vi "Read Waveform Measurement Two Channel.vi"(5 "Channel B (2: Channel 2)":u16(ring)=2 items=["Channel 1"=1, "Channel 2"=2, "Channel 3"=3, "Channel 4"=4], 6 "Measurement Function (0: Falling Edge)":u16(ring) items=["VRatio(Display)", "VRatio(Cycle)", "Raising Edge Delay", "Falling Edge Delay", "Raising to Falling Edge Delay", "Falling to Raising Edge Delay", "Raising Edge Phase", "Falling Edge Phase"], 7 "Channel A(1: Channel 1)":u16(ring)=1 items=["Channel 1"=1, "Channel 2"=2, "Channel 3"=3, "Channel 4"=4], 8 "error in (no error)":errorcluster, 9 "Measurement Type (0: Statistic Average)":u16(ring) items=["Statistic Average", "Current Statistic Value", "Statistic Maximum", "Statistic Minimum", "Statistic Standard Deviation", "Counter"], 10 "Timeout (1000 ms)":dbl=1000.0, 11 "VISA resource name":refnum<visa-resource-name>) -> (0 "error out":errorcluster, 2 "Measurement":dbl, 3 "VISA resource name out":refnum<visa-resource-name>)   [LabVIEW 2015, in "ZhiYuan ZDS Series for TCP.lvlib"]
doc: "Returns the waveform the oscilloscope acquired for the specified channel. The waveform is from an acquisition that you initiate prior to calling this VI.\n\nYou use the Initiate VI to start an acquisition on the channels that you enable with the Configure Channel VI. The oscilloscope acquires waveforms for the enabled channels concurrently. You must call this VI separately for each enabled channel to obtain the waveforms.\n\nYou can call the Read Waveform VI instead of using low-level VIs.\n\n<B>Note:</B> Use this VI only with other low-level VIs. The high-level VIs automatically incorporate this functionality. This VI does not check the instrument status."
uses:
  ZhiYuan ZDS Series for TCP.lvlib
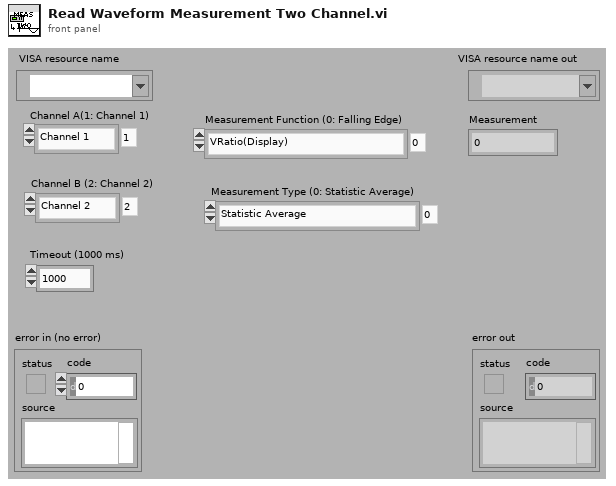
[diagram p1: front panel]
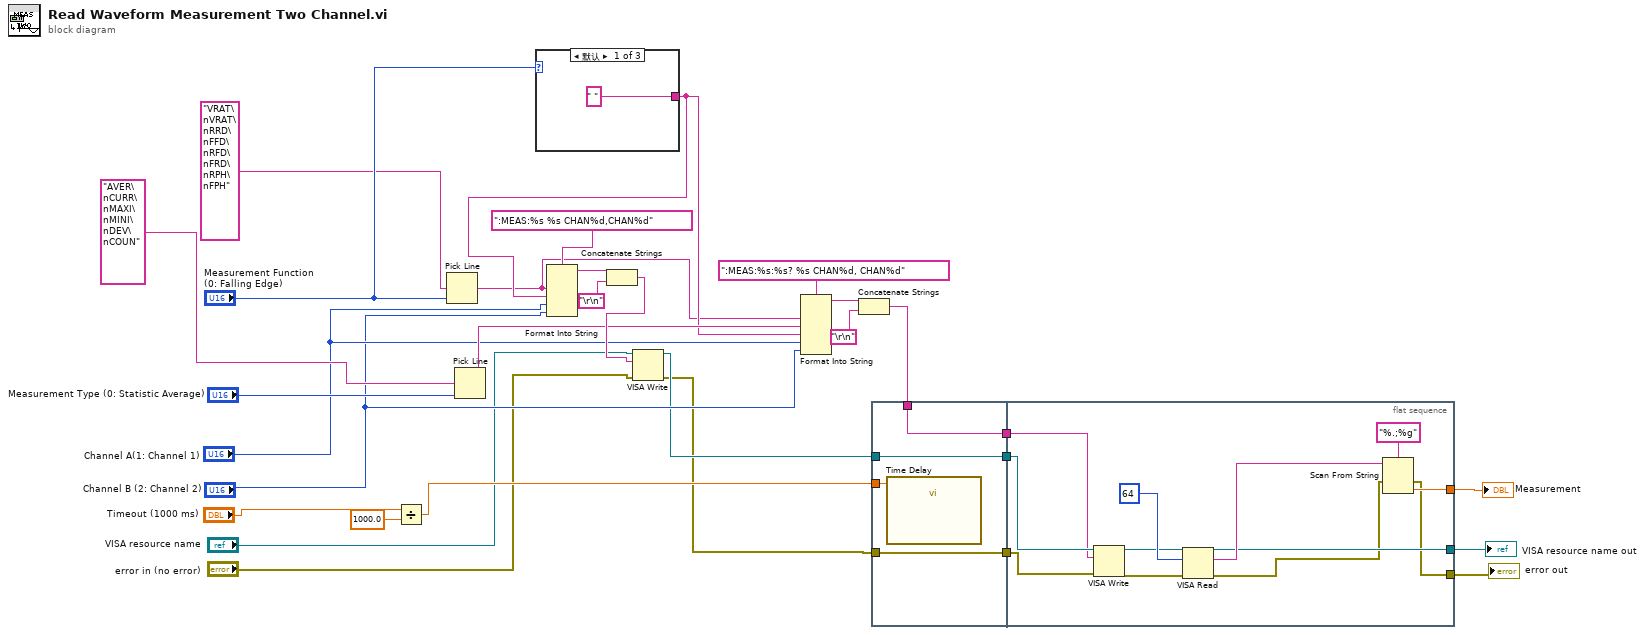
[diagram p0: block diagram]
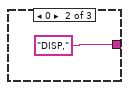
[diagram p2: hidden frame]
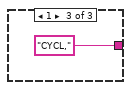
[diagram p3: hidden frame]
diagram:
  n1 = Divide(x="Timeout (1000 ms)", y=1000.0) -> (x/y=w10:dbl)
  n2 = Pick Line(multi-line string="VRAT\nVRAT\nRRD\nFFD\nRFD\nFRD\nRPH\nFPH", line index="Measurement Function (0: Falling Edge)") -> (output string=w1:string)  [unwired: 1 in]
  n3 = Pick Line(multi-line string="AVER\nCURR\nMAXI\nMINI\nDEV\nCOUN", line index="Measurement Type (0: Statistic Average)") -> (output string=w19:string)  [unwired: 1 in]
  n4 = case shown="默认" "Measurement Function (0: Falling Edge)" {
    tunnel: [" " "DISP," "CYCL,"] -> w18
    frame Default {
    }
    frame 0 {
    }
    frame 1 {
    }
  }
  n5 = Format Into String(format string=":MEAS:%s %s CHAN%d,CHAN%d" ("write buffer"), w1, w18, "Channel A(1: Channel 1)", "Channel B (2: Channel 2)") -> (resulting string=w24:string)  [unwired: 2 in, 1 out]
  n6 = Concatenate Strings(w24, "\r\n") -> (w22:string)
  n7 = VISA Write(VISA resource name="VISA resource name", write buffer=w22, error in (no error)="error in (no error)") -> (VISA resource name out=w3:refnum<visa-resource-name>, error out=w2:errorcluster)  [unwired: 1 out]
  n8 = Format Into String(format string=":MEAS:%s:%s? %s CHAN%d, CHAN%d", w1, w19, w18, "Channel A(1: Channel 1)", "Channel B (2: Channel 2)") -> (resulting string=w15:string)  [unwired: 2 in, 1 out]
  n9 = Concatenate Strings(w15, "\r\n") -> (w5:string)
  n10 = flat-sequence {
    tunnel: w10 -> [w37]
    tunnel: w3 -> [w36]
    tunnel: [w36] -> w8
    tunnel: [w35] -> w7
    tunnel: w2 -> [w35]
    tunnel: w5 -> [w34]
    tunnel: [w34] -> w4
    tunnel: [w45] -> w28
    tunnel: [w43] -> w21
    tunnel: [w41] -> w13
    tunnel: w8 -> [w40]
    tunnel: w7 -> [w39]
    tunnel: w4 -> [w38]
    frame #0 {
      n11 = call "Time Delay"("Delay Time (s)"=w37) -> ()  [unwired: 10 in, 1 out]
    }
    frame #1 {
      n12 = VISA Write(VISA resource name=w40, write buffer=w38, error in (no error)=w39) -> (VISA resource name out=w48:refnum<visa-resource-name>, error out=w47:errorcluster)  [unwired: 1 out]
      n13 = VISA Read(VISA resource name=w48, byte count=u32 64, error in (no error)=w47) -> (VISA resource name out=w43:refnum<visa-resource-name>, read buffer=w44:string, error out=w42:errorcluster)  [unwired: 1 out]
      n14 = Scan From String(format string="%.;%g", input string=w44, error in=w42) -> (error out=w41:errorcluster, output 1=w45:dbl)  [unwired: 2 in, 2 out]
    }
  }
  "error out" <- w13
  "VISA resource name out" <- w21
  "Measurement" <- w28
